vi "Close.vi"(8 "error in (no error)":errorcluster, 11 "NetworkStreamReader in":refnum<class "NetworkStreamReader.lvclass">) -> (0 "error out":errorcluster)   [LabVIEW 2013, in "NetworkStreamReader.lvclass"]
doc: "Properly closes a NetworkStreamReader Object.\n\n<b>It is critical that all initialized NetworkStreamReader Objects are closed with the Close method.</b> This method signals the background process to stop. If the Close method is not called, the background process will continue to run on the host computer. For this reason, <b>do not abort an application which uses NetworkStreamReader Objects.</b>\n\nJared Kirschner, 2012."
uses:
  NetworkStreamReader.lvclass
  NetworkStreamReader.lvclass/NetworkStreamReader.ctl
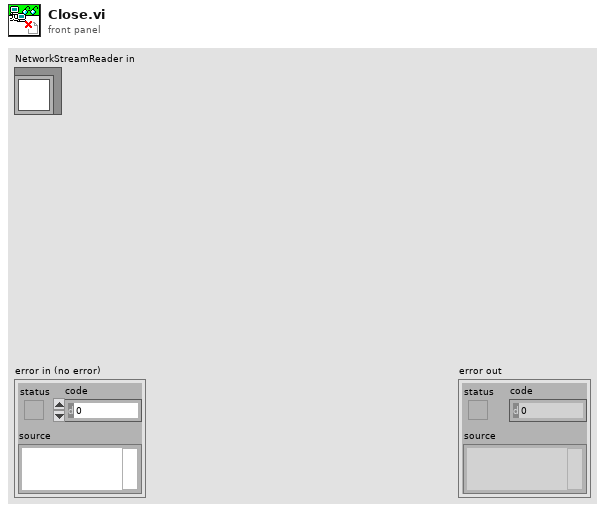
[diagram p1: front panel]
types:
  T1 = typedef "TimeStampedMessageQueue.ctl" = refnum<queue>
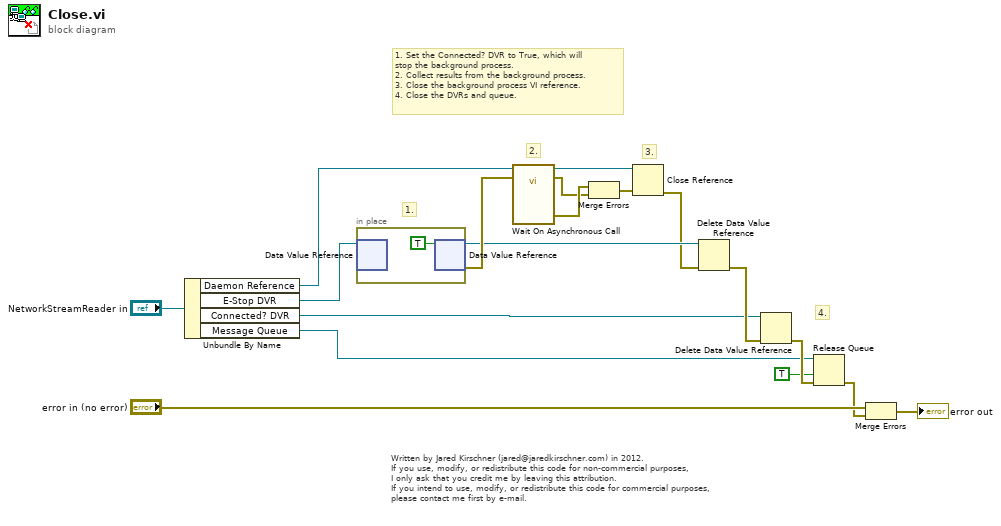
[diagram p0: block diagram]
diagram:
  # "4."
  # "3."
  # "2."
  # "1."
  # "1. Set the Connected? DVR to True, which will\nstop the background process.\n2. Collect results from the background process.\n3. Close the background process VI reference.\n4. Close the DVRs and queue."
  # "Written by Jared Kirschner (jared@jaredkirschner.com) in 2012.\nIf you use, modify, or redistribute this code for non-commercial purposes,\nI only ask that you credit me by leaving this attribution.\nIf you intend to use, modify, or redistribute this code for commercial purposes,\nplease contact me first by e-mail."
  n1 = Unbundle By Name("NetworkStreamReader in") -> ("Daemon Reference"=w12:refnum<vi>, "E-Stop DVR"=w6:refnum<data-value>, "Connected? DVR"=w5:refnum<data-value>, "Message Queue"=w2:T1)
  n2 = in-place {
    n3 = in-place-dvr #1(w6) -> ()  [unwired: 2 out]
    n4 = in-place-dvr #1(TRUE ("data value")) -> (w10:refnum<data-value>, w13:errorcluster)
  }
  n5 = call-by-ref "Wait On Asynchronous Call"(reference=w12, error in=w13) -> (reference out=w17:refnum<vi>, error out=w14:errorcluster, 0:"error out"=w15:errorcluster)  [unwired: 11 in]
  n6 = Merge Errors(w15, w14) -> (w16:errorcluster)
  n7 = Close Reference(reference=w17, error in (no error)=w16) -> (error out=w9:errorcluster)
  n8 = Delete Data Value Reference(data value reference=w10, error in=w9) -> (error out=w11:errorcluster)  [unwired: 1 out]
  n9 = Delete Data Value Reference(data value reference=w5, error in=w11) -> (error out=w3:errorcluster)  [unwired: 1 out]
  n10 = Release Queue(queue=w2, force destroy? (F)=TRUE, error in (no error)=w3) -> (error out=w4:errorcluster)  [unwired: 2 out]
  n11 = Merge Errors("error in (no error)", w4) -> (→"error out":errorcluster)
